vi "Configure Instrument Date Time.vi"(8 "error in (no error)":errorcluster, 10 "Time Stamp (0)":timestamp=timestamp(3029526000 s since 1904-01-01), 11 "VISA resource name":refnum<visa-resource-name>) -> (0 "error out":errorcluster, 3 "VISA resource name out":refnum<visa-resource-name>)   [LabVIEW 2017, in "HH PLI Series.lvlib"]
doc: "Configures the instrument date and time."
uses:
  HH PLI Series.lvlib
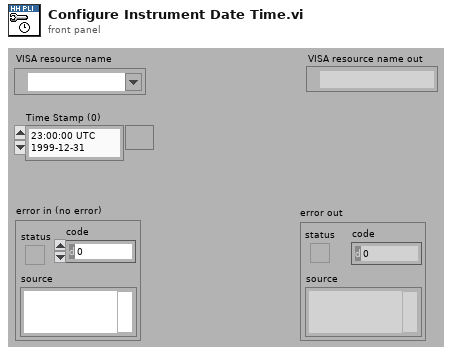
[diagram p1: front panel]
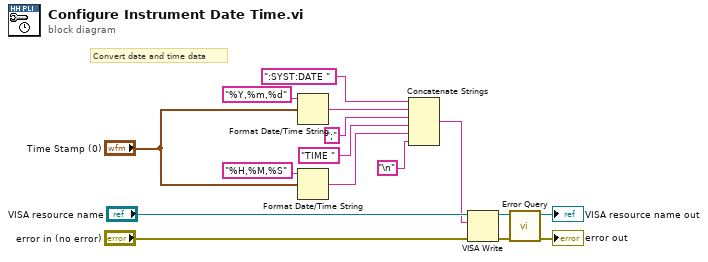
[diagram p0: block diagram]
diagram:
  # "Convert date and time data"
  n1 = Format Date/Time String(time format string (%c)="%Y,%m,%d", seconds (now)="Time Stamp (0)") -> (date/time string=w6:string)  [unwired: 1 in]
  n2 = Format Date/Time String(time format string (%c)="%H,%M,%S", seconds (now)="Time Stamp (0)") -> (date/time string=w3:string)  [unwired: 1 in]
  n3 = Concatenate Strings(":SYST:DATE " ("command"), w6, ";" ("string"), "TIME " ("string"), w3, "\n") -> (w1:string)
  n4 = VISA Write(VISA resource name="VISA resource name", write buffer=w1, error in (no error)="error in (no error)") -> (VISA resource name out=w14:refnum<visa-resource-name>, error out=w15:errorcluster)  [unwired: 1 out]
  n5 = call "Error Query.vi"("error in (no error)"=w15, "VISA resource name"=w14) -> ("error out"=→"error out":errorcluster, "VISA resource name out"=→"VISA resource name out":refnum<visa-resource-name>)  [unwired: 6 in, 2 out]
